vi "Z6_Beamline.PopUpBox.vi"(0 "node":string, 1 "systemID":string, 2 "instance":string) -> ()   [LabVIEW 2009]
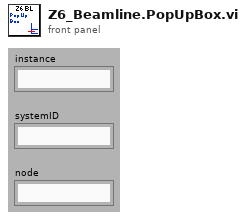
[diagram p1: front panel]
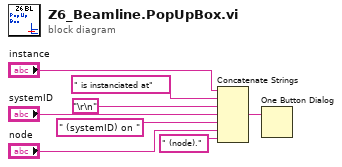
[diagram p0: block diagram]
diagram:
  n1 = Concatenate Strings("instance", " is instanciated at", "\r\n", "systemID", " (systemID) on ", "node", " (node).") -> (w8:string)
  n2 = One Button Dialog(message=w8) -> ()  [unwired: 1 in, 1 out]
